vi "手势匹配.vi"(0 "源图片":T1, 1 "上":T1, 2 "下":T1, 3 "左":T1, 4 "右":T1, 5 "最小匹配度":sgl=500.0, 6 "匹配算法0":i32(ring)=2 items=["All", "Low Discrepancy Sampling", "Grayscale Value Pyramid", "Gradients Pyramid"], 7 "匹配参数0":T3={"Number of Matches Requested"=1, "Minimum Match Score"=750.0, "Angle Ranges"=[]} {"Angle Ranges"."End Angle" min=-360 max=360; "Angle Ranges"."Start Angle" min=-360 max=360; "Minimum Match Score" min=0 max=1000; "Number of Matches Requested" min=1 max=9999}, 8 "匹配算法1":i32(ring)=2 items=["All", "Low Discrepancy Sampling", "Grayscale Value Pyramid", "Gradients Pyramid"], 9 "匹配参数1":T3={"Number of Matches Requested"=1, "Minimum Match Score"=750.0, "Angle Ranges"=[]} {"Angle Ranges"."End Angle" min=-360 max=360; "Angle Ranges"."Start Angle" min=-360 max=360; "Minimum Match Score" min=0 max=1000; "Number of Matches Requested" min=1 max=9999}, 10 "匹配算法2":i32(ring)=2 items=["All", "Low Discrepancy Sampling", "Grayscale Value Pyramid", "Gradients Pyramid"], 11 "匹配参数2":T3={"Number of Matches Requested"=1, "Minimum Match Score"=750.0, "Angle Ranges"=[]} {"Angle Ranges"."End Angle" min=-360 max=360; "Angle Ranges"."Start Angle" min=-360 max=360; "Minimum Match Score" min=0 max=1000; "Number of Matches Requested" min=1 max=9999}, 12 "匹配算法3":i32(ring)=2 items=["All", "Low Discrepancy Sampling", "Grayscale Value Pyramid", "Gradients Pyramid"], 13 "匹配参数3":T3={"Number of Matches Requested"=1, "Minimum Match Score"=750.0, "Angle Ranges"=[]} {"Angle Ranges"."End Angle" min=-360 max=360; "Angle Ranges"."Start Angle" min=-360 max=360; "Minimum Match Score" min=0 max=1000; "Number of Matches Requested" min=1 max=9999}) -> (14 "输出图":T1(plugin-control), 19 "结果":i32)   [LabVIEW 2014]
uses:
  <vilib>/vision/Image Controls.llb/IMAQ Image.ctl
  <vilib>/vision/NI_Vision_Development_Module.lvlib
panel:
  out "3 2":T1(plugin-control)
  out "2 2":T1(plugin-control)
  out "1 2":T1(plugin-control)
  out "0 2":T1(plugin-control)
  out "3":T1(plugin-control)
  out "2":T1(plugin-control)
  out "1":T1(plugin-control)
  out "0":T1(plugin-control)
  out "源":T1(plugin-control)
  out "匹配结果3":T2(array[cluster]) {"Bounding Box"."y" format="%.2g"; "Bounding Box"."x" format="%.2g"; "Score" format="%.2f"; "Scale" format="%.2g"; "Angle" format="%.2g"; "Position"."y" format="%.2g"; "Position"."x" format="%.2g"}
  in  "高级选项3":cluster{"Item":u16, "Value":dbl}[](array[cluster])=[{"Item"=1, "Value"=1.0}, {"Item"=103, "Value"=1.0}] {"Item" items=["LD Sampling - Minimum Constrast"=0, "LD Sampling - Enable Subpixel Accuracy"=1, "LD Sampling - Search Strategy"=2, "LD Sampling - Subpixel Iterations"=3, "LD Sampling - Subpixel Tolerance"=4, "LD Sampling - Initial Match List Length"=5, "LD Sampling - Match List Reduction Factor"=6, "LD Sampling - Initial Step Size"=7, "LD Sampling - Intermediate Angular Accuracy"=8, "-"=9, "Pyramid - Max Pyramid Level"=100, "Pyramid - Minimum Contrast"=102, "Pyramid - Enable Subpixel Accuracy"=103, "Pyramid - Subpixel Iterations"=104, "Pyramid - Subpixel Tolerance"=105, "Pyramid - Initial Match List Length"=106, "Pyramid - Match List Reduction Factor"=107, "Pyramid - Intermediate Angular Accuracy"=108, "Pyramid - Process Border Matches"=109, "Pyramid - Min Match Separation Distance"=111, "Pyramid - Min Match Separation Angle"=112, "Pyramid - Max Match Overlap"=113, "Pyramid - Max Cache in MB"=114, "Pyramid - Clear Cache"=115]}
  out "找到的数量3":i32
  out "匹配结果2":T2(array[cluster]) {"Bounding Box"."y" format="%.2g"; "Bounding Box"."x" format="%.2g"; "Score" format="%.2f"; "Scale" format="%.2g"; "Angle" format="%.2g"; "Position"."y" format="%.2g"; "Position"."x" format="%.2g"}
  in  "高级选项2":cluster{"Item":u16, "Value":dbl}[](array[cluster])=[{"Item"=1, "Value"=1.0}, {"Item"=103, "Value"=1.0}] {"Item" items=["LD Sampling - Minimum Constrast"=0, "LD Sampling - Enable Subpixel Accuracy"=1, "LD Sampling - Search Strategy"=2, "LD Sampling - Subpixel Iterations"=3, "LD Sampling - Subpixel Tolerance"=4, "LD Sampling - Initial Match List Length"=5, "LD Sampling - Match List Reduction Factor"=6, "LD Sampling - Initial Step Size"=7, "LD Sampling - Intermediate Angular Accuracy"=8, "-"=9, "Pyramid - Max Pyramid Level"=100, "Pyramid - Minimum Contrast"=102, "Pyramid - Enable Subpixel Accuracy"=103, "Pyramid - Subpixel Iterations"=104, "Pyramid - Subpixel Tolerance"=105, "Pyramid - Initial Match List Length"=106, "Pyramid - Match List Reduction Factor"=107, "Pyramid - Intermediate Angular Accuracy"=108, "Pyramid - Process Border Matches"=109, "Pyramid - Min Match Separation Distance"=111, "Pyramid - Min Match Separation Angle"=112, "Pyramid - Max Match Overlap"=113, "Pyramid - Max Cache in MB"=114, "Pyramid - Clear Cache"=115]}
  out "找到的数量2":i32
  out "匹配结果1":T2(array[cluster]) {"Bounding Box"."y" format="%.2g"; "Bounding Box"."x" format="%.2g"; "Score" format="%.2f"; "Scale" format="%.2g"; "Angle" format="%.2g"; "Position"."y" format="%.2g"; "Position"."x" format="%.2g"}
  in  "高级选项1":cluster{"Item":u16, "Value":dbl}[](array[cluster])=[{"Item"=1, "Value"=1.0}, {"Item"=103, "Value"=1.0}] {"Item" items=["LD Sampling - Minimum Constrast"=0, "LD Sampling - Enable Subpixel Accuracy"=1, "LD Sampling - Search Strategy"=2, "LD Sampling - Subpixel Iterations"=3, "LD Sampling - Subpixel Tolerance"=4, "LD Sampling - Initial Match List Length"=5, "LD Sampling - Match List Reduction Factor"=6, "LD Sampling - Initial Step Size"=7, "LD Sampling - Intermediate Angular Accuracy"=8, "-"=9, "Pyramid - Max Pyramid Level"=100, "Pyramid - Minimum Contrast"=102, "Pyramid - Enable Subpixel Accuracy"=103, "Pyramid - Subpixel Iterations"=104, "Pyramid - Subpixel Tolerance"=105, "Pyramid - Initial Match List Length"=106, "Pyramid - Match List Reduction Factor"=107, "Pyramid - Intermediate Angular Accuracy"=108, "Pyramid - Process Border Matches"=109, "Pyramid - Min Match Separation Distance"=111, "Pyramid - Min Match Separation Angle"=112, "Pyramid - Max Match Overlap"=113, "Pyramid - Max Cache in MB"=114, "Pyramid - Clear Cache"=115]}
  out "找到的数量1":i32
  out "找到的数量0":i32
  in  "高级选项0":cluster{"Item":u16, "Value":dbl}[](array[cluster])=[{"Item"=1, "Value"=1.0}, {"Item"=103, "Value"=1.0}] {"Item" items=["LD Sampling - Minimum Constrast"=0, "LD Sampling - Enable Subpixel Accuracy"=1, "LD Sampling - Search Strategy"=2, "LD Sampling - Subpixel Iterations"=3, "LD Sampling - Subpixel Tolerance"=4, "LD Sampling - Initial Match List Length"=5, "LD Sampling - Match List Reduction Factor"=6, "LD Sampling - Initial Step Size"=7, "LD Sampling - Intermediate Angular Accuracy"=8, "-"=9, "Pyramid - Max Pyramid Level"=100, "Pyramid - Minimum Contrast"=102, "Pyramid - Enable Subpixel Accuracy"=103, "Pyramid - Subpixel Iterations"=104, "Pyramid - Subpixel Tolerance"=105, "Pyramid - Initial Match List Length"=106, "Pyramid - Match List Reduction Factor"=107, "Pyramid - Intermediate Angular Accuracy"=108, "Pyramid - Process Border Matches"=109, "Pyramid - Min Match Separation Distance"=111, "Pyramid - Min Match Separation Angle"=112, "Pyramid - Max Match Overlap"=113, "Pyramid - Max Cache in MB"=114, "Pyramid - Clear Cache"=115]}
  out "匹配结果0":T2(array[cluster]) {"Bounding Box"."y" format="%.2g"; "Bounding Box"."x" format="%.2g"; "Score" format="%.2f"; "Scale" format="%.2g"; "Angle" format="%.2g"; "Position"."y" format="%.2g"; "Position"."x" format="%.2g"}
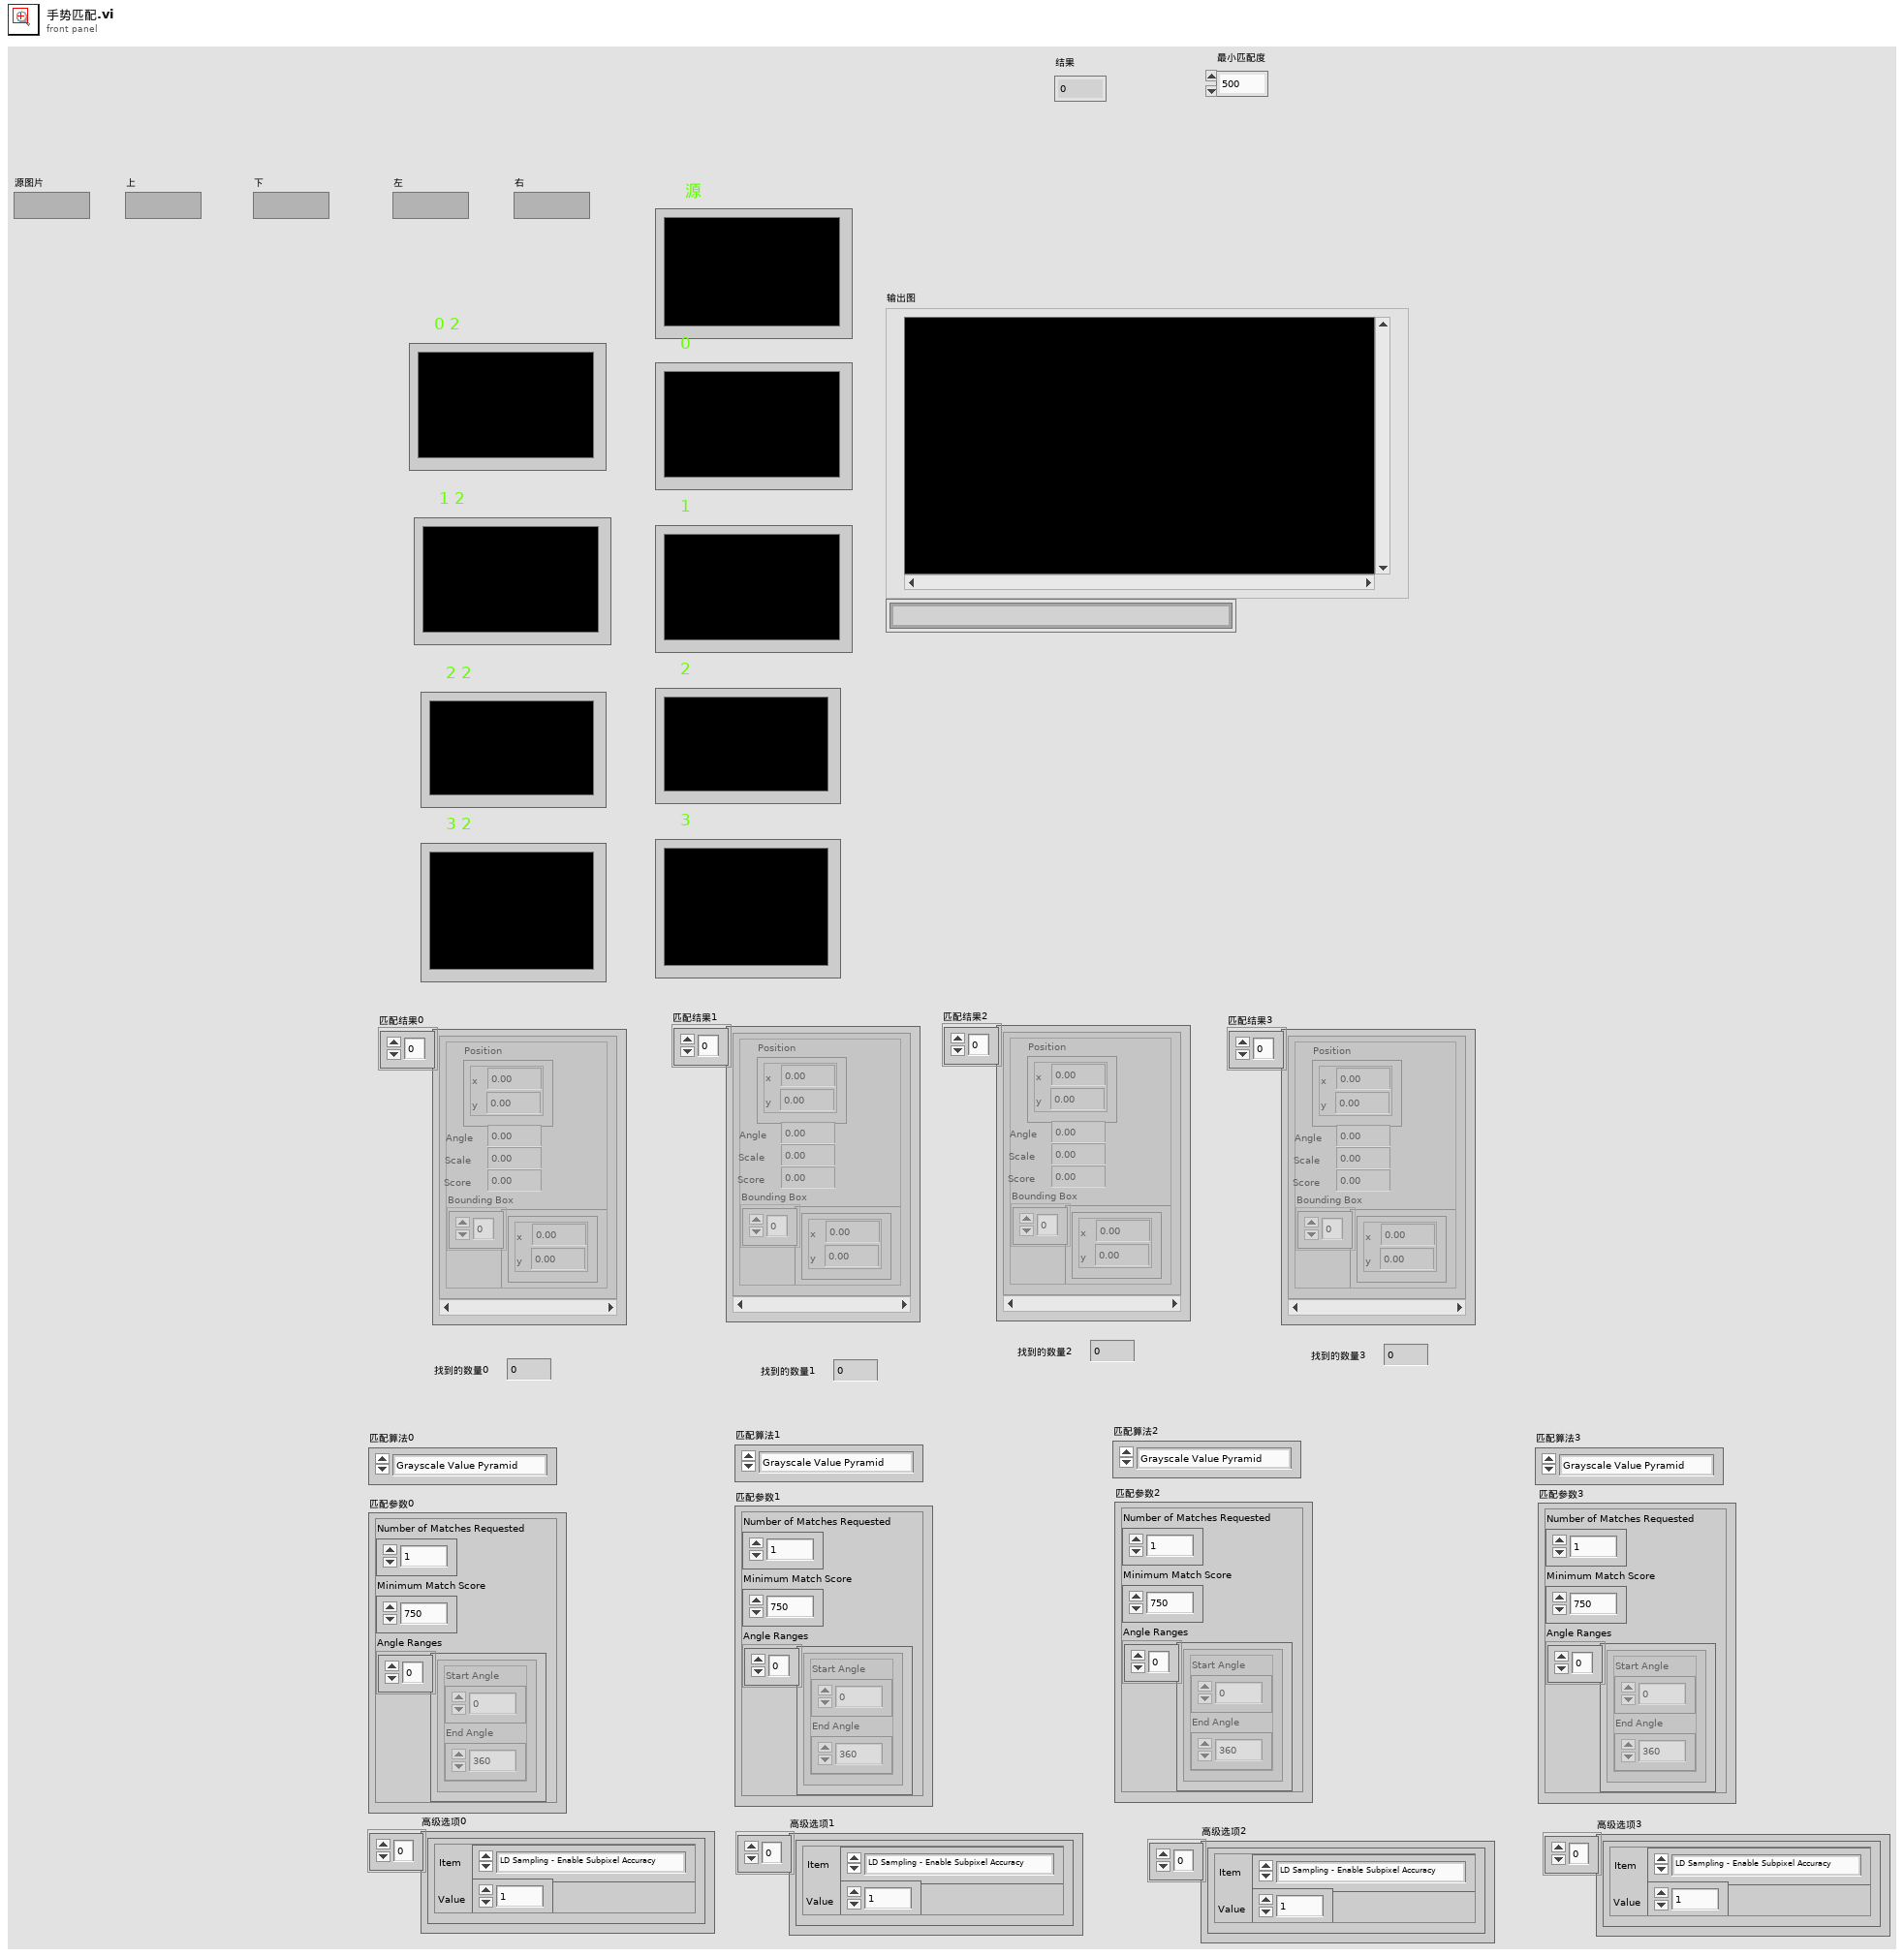
[diagram p1: front panel]
types:
  T1 = typedef "IMAQ Image.ctl" = refnum<image>
  T2 = cluster{"Position":cluster{"x":sgl, "y":sgl}, "Angle":sgl, "Scale":sgl, "Score":sgl, "Bounding Box":cluster{"x":sgl, "y":sgl}[]}[]
  T3 = cluster{"Number of Matches Requested":i32, "Minimum Match Score":sgl, "Angle Ranges":cluster{"Start Angle":sgl, "End Angle":sgl}[]}
  T4 = typedef "Image Type" = u32
  T5 = cluster{"Position":cluster{"x":sgl, "y":sgl}, "Angle":sgl, "Scale":sgl, "Score":sgl, "Bounding Box":cluster{"x":sgl, "y":sgl}[]}
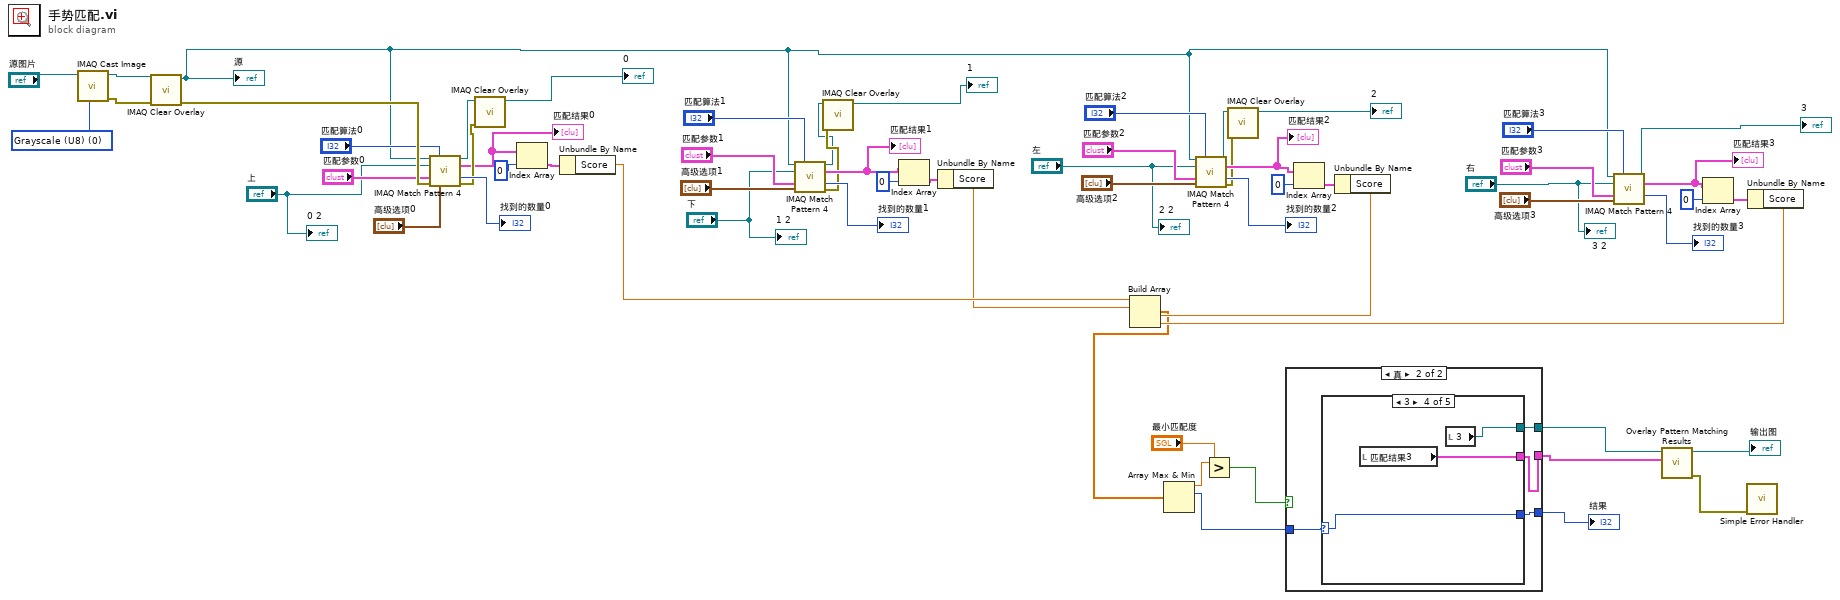
[diagram p0: block diagram]
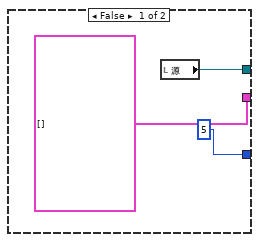
[diagram p2: hidden frame]
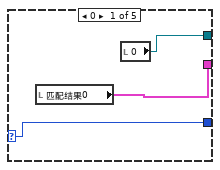
[diagram p3: hidden frame]
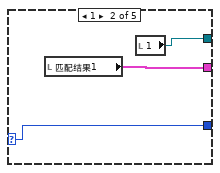
[diagram p4: hidden frame]
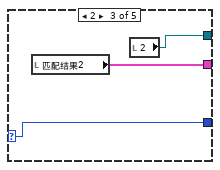
[diagram p5: hidden frame]
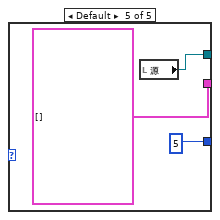
[diagram p6: hidden frame]
diagram:
  w59 = T4 0 items=["Grayscale (U8)", "Grayscale (I16)", "Grayscale (SGL)", "Complex (CSG)", "RGB (U32)", "HSL (U32)", "RGB (U64)", "Grayscale (U16)"] ("Image Type")
  n1 = call "IMAQ Cast Image"("Image Type"=w59, "Image Src"="源图片") -> ("error out"=w57:errorcluster, "Image Dst Out"=w56:T1)  [unwired: 8 in]
  n2 = call "IMAQ Clear Overlay"("error in (no error)"=w57, "Image"=w56) -> ("error out"=w54:errorcluster, "Image Out"=w6:T1)  [unwired: 8 in]
  "源" <- w6
  n3 = call "IMAQ Match Pattern 4"("Image"=w6, "Algorithm"="匹配算法0", "Template Image"="上", "Parameters"="匹配参数0", "error in (no error)"=w54, "Advanced Options"="高级选项0") -> ("Image (duplicate)"=w14:T1, "Matches (pixel)"=w10:T2, "Number of Matches"=→"找到的数量0":i32, "error out"=w15:errorcluster)  [unwired: 5 in, 1 out]
  "匹配结果0" <- w10
  n4 = call "IMAQ Clear Overlay"("error in (no error)"=w15, "Image"=w14) -> ("Image Out"=→"0":T1)  [unwired: 8 in, 1 out]
  n5 = Index Array(array=w10, index=0 ("索引")) -> (element=w11:T5)
  n6 = Unbundle By Name(w11) -> ("Score"=w53:sgl)
  n7 = call "IMAQ Match Pattern 4"("Image"=w6, "Algorithm"="匹配算法1", "Template Image"="下", "Parameters"="匹配参数1", "Advanced Options"="高级选项1") -> ("Image (duplicate)"=w13:T1, "Matches (pixel)"=w35:T2, "Number of Matches"=→"找到的数量1":i32, "error out"=w16:errorcluster)  [unwired: 6 in, 1 out]
  "匹配结果1" <- w35
  n8 = call "IMAQ Clear Overlay"("error in (no error)"=w16, "Image"=w13) -> ("Image Out"=→"1":T1)  [unwired: 8 in, 1 out]
  n9 = Index Array(array=w35, index=0 ("索引")) -> (element=w41:T5)
  n10 = Unbundle By Name(w41) -> ("Score"=w52:sgl)
  n11 = call "IMAQ Match Pattern 4"("Image"=w6, "Algorithm"="匹配算法2", "Template Image"="左", "Parameters"="匹配参数2", "Advanced Options"="高级选项2") -> ("Image (duplicate)"=w12:T1, "Matches (pixel)"=w27:T2, "Number of Matches"=→"找到的数量2":i32, "error out"=w17:errorcluster)  [unwired: 6 in, 1 out]
  "匹配结果2" <- w27
  n12 = call "IMAQ Clear Overlay"("error in (no error)"=w17, "Image"=w12) -> ("Image Out"=→"2":T1)  [unwired: 8 in, 1 out]
  n13 = Index Array(array=w27, index=0 ("索引")) -> (element=w33:T5)
  n14 = Unbundle By Name(w33) -> ("Score"=w51:sgl)
  n15 = call "IMAQ Match Pattern 4"("Image"=w6, "Algorithm"="匹配算法3", "Template Image"="右", "Parameters"="匹配参数3", "Advanced Options"="高级选项3") -> ("Image (duplicate)"=→"3":T1, "Matches (pixel)"=w19:T2, "Number of Matches"=→"找到的数量3":i32)  [unwired: 6 in, 2 out]
  "匹配结果3" <- w19
  n16 = Index Array(array=w19, index=0 ("索引")) -> (element=w25:T5)
  n17 = Unbundle By Name(w25) -> ("Score"=w50:sgl)
  n18 = Build Array(w53, w52, w51, w50) -> (w48:sgl[])
  n19 = Array Max & Min(array=w48) -> (max value=w62:sgl, max index (indices)=w60:i32)  [unwired: 2 out]
  n20 = Greater?(x=w62, y="最小匹配度") -> (0:w61:bool)
  n21 = case shown="真" w61 {
    tunnel: w60 -> [_ w69]
    tunnel: [5 w68] -> w49
    tunnel: [T2 [] ("匹配结果3") w67] -> w7
    tunnel: [w63 w66] -> w5
    frame False {
      n22 = local read "源"() -> (w63:T1)
    }
    frame True {
      n23 = case shown="3" w69 {
        selector: w69 -> [w72 w75 w78 w81 _]
        tunnel: [w72 w75 w78 w81 5] -> w68
        tunnel: [w71 w74 w77 w80 T2 [] ("匹配结果3")] -> w67
        tunnel: [w70 w73 w76 w79 w82] -> w66
        frame 0 {
          n24 = local read "匹配结果0"() -> (w71:T2)
          n25 = local read "0"() -> (w70:T1)
        }
        frame 1 {
          n26 = local read "匹配结果1"() -> (w74:T2)
          n27 = local read "1"() -> (w73:T1)
        }
        frame 2 {
          n28 = local read "匹配结果2"() -> (w77:T2)
          n29 = local read "2"() -> (w76:T1)
        }
        frame 3 {
          n30 = local read "匹配结果3"() -> (w80:T2)
          n31 = local read "3"() -> (w79:T1)
        }
        frame Default {
          n32 = local read "源"() -> (w82:T1)
        }
      }
    }
  }
  "结果" <- w49
  n33 = call "Overlay Pattern Matching Results.vi"("Matches"=w7, "Image"=w5) -> ("error out"=w8:errorcluster, "Image Out"=→"输出图":T1)  [unwired: 8 in]
  n34 = call <vilib>:"Simple Error Handler.vi"("error in (no error)"=w8) -> ()  [unwired: 4 in, 5 out]
  "0 2" <- "上"
  "1 2" <- "下"
  "2 2" <- "左"
  "3 2" <- "右"
